vi "Actor Core.vi"(8 "error in":errorcluster, 11 "Root Panel Actor in":refnum<class "Root Panel Actor.lvclass">) -> (0 "error out":errorcluster, 3 "Actor out":refnum<class "Actor.lvclass">)   [LabVIEW 2021, in "Root Panel.lvlib" / "Root Panel Actor.lvclass"]
doc: "The user interface for this panel.\n\n----\nPlease see the following web address for additional documentation and tutorial information:\nhttp://www.mooregoodideas.com/mgi-panel-manager/\n\nAuthor: Derek Trepanier\n\nCopyright (c) 2018, Moore Good Ideas, Inc.\n\nAll rights reserved.\n\nRedistribution and use in source and binary forms, with or without modification, are permitted provided that the following conditions are met:\n\n * Redistributions of source code must retain the above copyright notice, this list of conditions and the following disclaimer.\n * Redistributions in binary form must reproduce the above copyright notice, this list of conditions and the following disclaimer in the documentation and/or other materials provided with the distribution.\n * Neither the name of Moore Good Ideas, Inc. nor the names of its contributors may be used to endorse or promote products derived from this software without specific prior written permission.\n\nTHIS SOFTWARE IS PROVIDED BY THE COPYRIGHT HOLDERS AND CONTRIBUTORS \"AS IS\" AND ANY EXPRESS OR IMPLIED WARRANTIES, INCLUDING, BUT NOT LIMITED TO, THE IMPLIED WARRANTIES OF MERCHANTABILITY AND FITNESS FOR A PARTICULAR PURPOSE ARE DISCLAIMED. IN NO EVENT SHALL THE COPYRIGHT OWNER OR CONTRIBUTORS BE LIABLE FOR ANY DIRECT, INDIRECT, INCIDENTAL, SPECIAL, EXEMPLARY, OR CONSEQUENTIAL DAMAGES (INCLUDING, BUT NOT LIMITED TO, PROCUREMENT OF SUBSTITUTE GOODS OR SERVICES; LOSS OF USE, DATA, OR PROFITS; OR BUSINESS INTERRUPTION) HOWEVER CAUSED AND ON ANY THEORY OF LIABILITY, WHETHER IN CONTRACT, STRICT LIABILITY, OR TORT (INCLUDING NEGLIGENCE OR OTHERWISE) ARISING IN ANY WAY OUT OF THE USE OF THIS SOFTWARE, EVEN IF ADVISED OF THE POSSIBILITY OF SUCH DAMAGE."
uses:
  Root Panel Actor.lvclass
  C:/Program Files (x86)/National Instruments/LabVIEW 2021/vi.lib/MGI/Panel Manager/Panel Actor/Panel Actor/Panel Actor.lvclass
  <vilib>/ActorFramework/Actor/Actor.lvclass
  Root Panel Actor.lvclass/Root Panel Actor.ctl
  <vilib>/ActorFramework/Message Enqueuer/Message Enqueuer.lvclass/Message Enqueuer.ctl
  Appearance Actor/Appearance Actor/Typedefs/User Event-Panel Resize-Data--cluster.ctl
  <vilib>/Utility/miscctls.llb/LVRectTypeDef.ctl
  <vilib>/event_ctls.llb/sizeaction.ctl
  <vilib>/event_ctls.llb/panelstate.ctl
  Appearance Actor/Appearance Actor Messages/User Event-Panel Resize Msg/User Event-Panel Resize Msg.lvclass/User Event-Panel Resize Msg.ctl
  <vilib>/ActorFramework/Message Enqueuer/Enqueue.vi
  <vilib>/ActorFramework/Stop Msg/Stop Msg.lvclass
  C:/Program Files (x86)/National Instruments/LabVIEW 2021/vi.lib/ActorFramework/Message/Message.lvclass
  Appearance Actor/Appearance Actor Messages/User Event-Close-Value Change Msg/User Event-Close-Value Change Msg.lvclass
  Appearance Actor/Appearance Actor Messages/User Event-Maximize-Value Change Msg/User Event-Maximize-Value Change Msg.lvclass
  Appearance Actor/Appearance Actor Messages/User Event-Minimize-Value Change Msg/User Event-Minimize-Value Change Msg.lvclass
  Appearance Actor/Appearance Actor Messages/User Event-Settings-Value Change Msg/User Event-Settings-Value Change Msg.lvclass
  Appearance Actor/Appearance Actor Messages/User Event-Title Bar-Mouse Down Msg/User Event-Title Bar-Mouse Down Msg.lvclass
  Appearance Actor/Appearance Actor Messages/User Event-Panel Resize Msg/User Event-Panel Resize Msg.lvclass
  <vilib>/ActorFramework/Message Priority Queue/Priority Enqueue.vi
  Appearance Actor/Appearance Actor/Appearance Actor.lvclass
  <vilib>/MGI/Panel Manager/Panel Actor/Panel Actor/Panel Actor.lvclass
  <vilib>/MGI/Panel Manager/Panel Actor/Panel Actor Messages/Show Panel Msg/Show Panel Msg.lvclass
  <vilib>/Thomas ALLIBE/Path Utilities/Path Utilities.lvlib
panel:
  in  "Title Bar L":bool
  out "App Icon":picture
  in  "Title Bar M":bool
  out "TB.Title":string
  in  "TB.Dark-Button.Maximize":bool
  in  "TB.Light-Button.Maximize":bool
  in  "TB.Dark-CloseButton":bool
  in  "TB.Light-CloseButton":bool
  in  "TB.Dark-Button.Minimize":bool
  in  "TB.Light-Button.Minimize":bool
  in  "Title Bar R":bool
  in  "SM.Dark-Button.Settings":bool
  in  "SM.Light-Button.Settings":bool
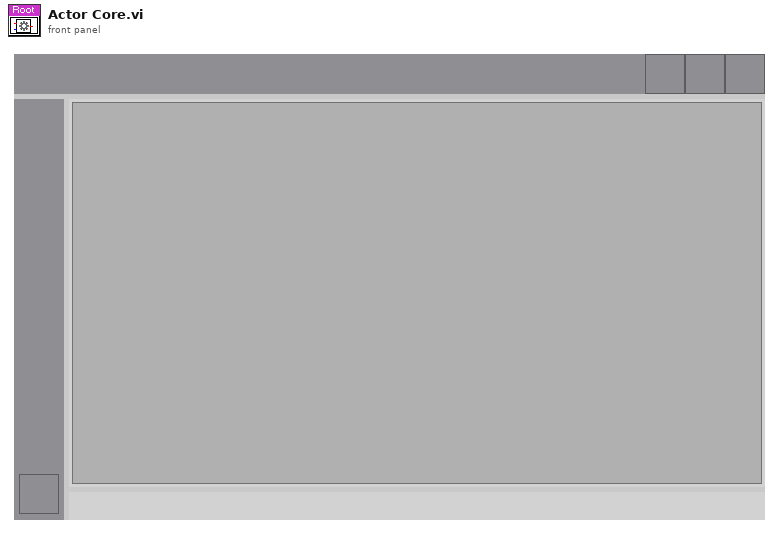
[diagram p1: front panel]
types:
  T1 = cluster{"left":i16, "top":i16, "right":i16, "bottom":i16}
  T2 = typedef "Appearance Actor.lvlib/Appearance Actor.lvclass/User Event-Panel Resize-Data--cluster.ctl" = cluster{"OldBnds":T3, "NewBnds":T3, "Act":T4, "PrevState":T5}
  T3 = typedef "LVRectTypeDef.ctl" = cluster{"Left":i16, "Top":i16, "Right":i16, "Bottom":i16}
  T4 = typedef "sizeaction.ctl" = enum32{"Minimized", "Maximized", "Resized"}
  T5 = typedef "panelstate.ctl" = enum32{"Standard", "Minimized", "Maximized"}
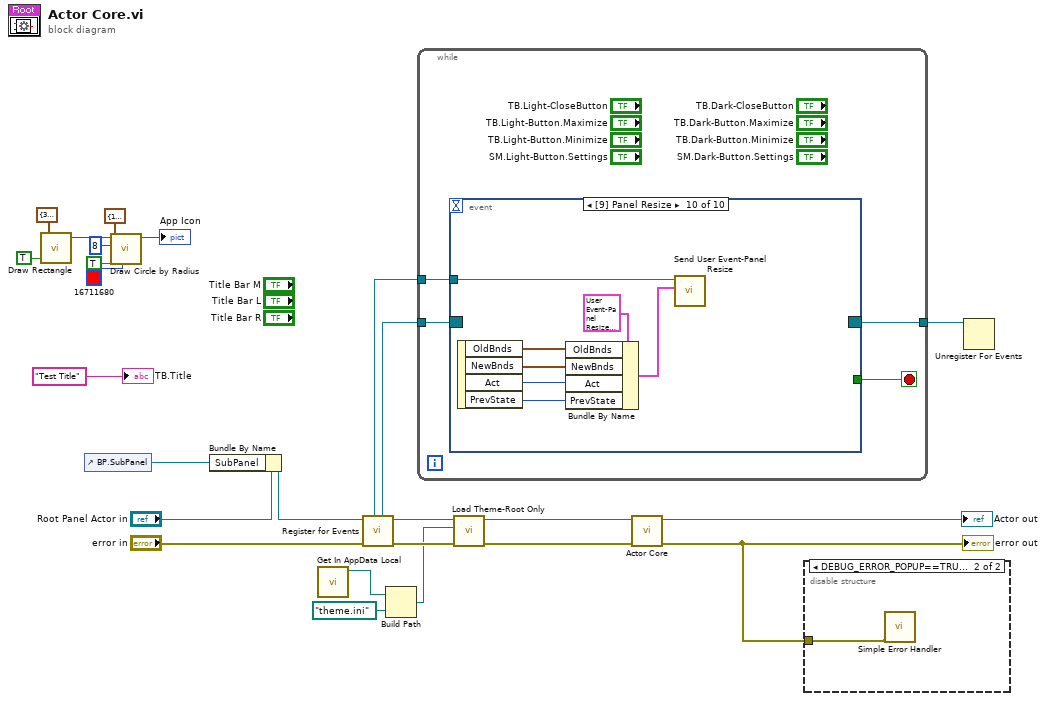
[diagram p0: block diagram]
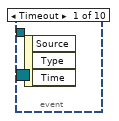
[diagram p3: hidden frame]
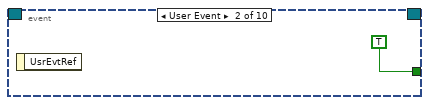
[diagram p4: hidden frame]
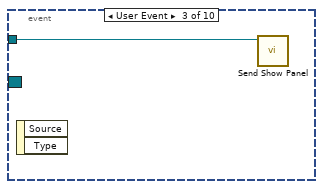
[diagram p5: hidden frame]
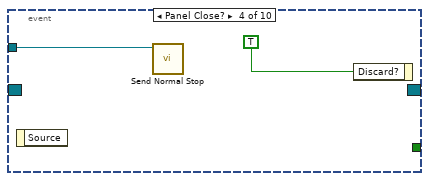
[diagram p6: hidden frame]
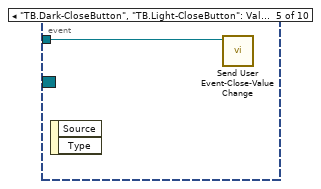
[diagram p7: hidden frame]
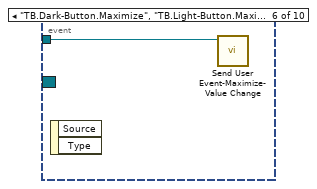
[diagram p8: hidden frame]
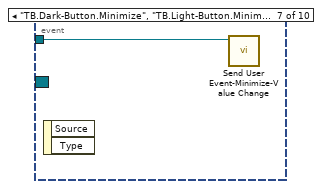
[diagram p9: hidden frame]
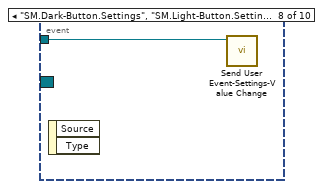
[diagram p10: hidden frame]
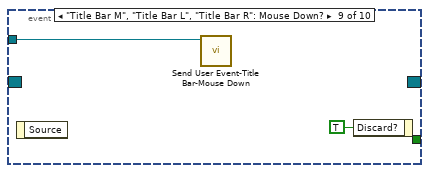
[diagram p11: hidden frame]
diagram:
  n1 = call <vilib>:"Draw Rectangle.vi"("rect"=T1 {"left"=3, "top"=3, "right"=40, "bottom"=30}, "fill?(F)"=TRUE) -> ("new picture"=w19:picture)  [unwired: 7 in]
  n2 = control-ref of="BP.SubPanel"() -> (w2:refnum<vi>)
  n3 = call <vilib>:"Draw Circle by Radius.vi"("color(black)"=u32 16711680, "fill?(F)"=TRUE, "pixel center"=cluster{"horizontal":i16, "vertical":i16} {"horizontal"=15, "vertical"=12}, "radius"=i16 8, "picture"=w19) -> ("new picture"=→"App Icon":picture)  [unwired: 6 in]
  n4 = Bundle By Name(cluster="Root Panel Actor in", "SubPanel"=w2) -> (w4:refnum<class "Root Panel Actor.lvclass">)
  n5 = call <vilib>:"Get In AppData Local.vi"() -> ("Path"=w9:path)  [unwired: 10 in, 1 out]
  n6 = call <vilib>:"Register for Events.vi"("Error In"="error in", "Panel Actor in"=w4) -> ("Error Out"=w11:errorcluster, "Panel Actor out"=w12:refnum<class "Root Panel Actor.lvclass">, "Pnl Actor"=w22:refnum<event-registration>, "Self Enqueuer"=w23:refnum<class "Message Enqueuer.lvclass">)  [unwired: 6 in]
  n7 = Build Path(base path=w9, name or relative path=path "theme.ini") -> (appended path=w7:path)
  n8 = while {
    tunnel: w22 -> [w29]
    tunnel: w23 -> [w28]
    tunnel: [w26] -> w24
    stop <- w27 stop-if-true
    n9 = event shown="[9] Panel Resize" {
      selector: w29 -> [_ _ _ _ _ _ _ _ _ _]
      dyn-events: [_ _ _ _ _ _ _ _ _ _] -> w26
      timeout: _ -> [_ _ _ _ _ _ _ _ _ _]
      tunnel: w28 -> [_ _ w31 w33 w34 w35 w36 w37 w38 w40]
      tunnel: [_ TRUE _ _ _ _ _ _ _ _] -> w27
      event Timeout {
        n10 = event-data() -> ()  [unwired: 1 in, 3 out]
      }
      event User Event {
        n11 = event-data() -> ()  [unwired: 1 in, 1 out]
      }
      event User Event {
        n12 = event-data() -> ()  [unwired: 1 in, 2 out]
        n13 = call <vilib>:"Send Show Panel.vi"("Message Enqueuer in"=w31) -> ()  [unwired: 9 in, 2 out]
      }
      event Panel Close? {
        n14 = event-data() -> ()  [unwired: 1 in, 1 out]
        n15 = call <vilib>:"Send Normal Stop.vi"("Message Enqueuer"=w33) -> ()  [unwired: 10 in, 1 out]
        n16 = event-data("Discard?"=TRUE) -> ()  [unwired: 1 in, 1 out]
      }
      event "TB.Dark-CloseButton", "TB.Light-CloseButton": Value Change {
        n17 = event-data() -> ()  [unwired: 1 in, 2 out]
        n18 = call "Send User Event-Close-Value Change.vi"("Message Enqueuer"=w34) -> ()  [unwired: 9 in, 2 out]
      }
      event "TB.Dark-Button.Maximize", "TB.Light-Button.Maximize": Value Change {
        n19 = event-data() -> ()  [unwired: 1 in, 2 out]
        n20 = call "Send User Event-Maximize-Value Change.vi"("Message Enqueuer"=w35) -> ()  [unwired: 9 in, 2 out]
      }
      event "TB.Dark-Button.Minimize", "TB.Light-Button.Minimize": Value Change {
        n21 = event-data() -> ()  [unwired: 1 in, 2 out]
        n22 = call "Send User Event-Minimize-Value Change.vi"("Message Enqueuer"=w36) -> ()  [unwired: 9 in, 2 out]
      }
      event "SM.Dark-Button.Settings", "SM.Light-Button.Settings": Value Change {
        n23 = event-data() -> ()  [unwired: 1 in, 2 out]
        n24 = call "Send User Event-Settings-Value Change.vi"("Message Enqueuer"=w37) -> ()  [unwired: 9 in, 2 out]
      }
      event "Title Bar M", "Title Bar L", "Title Bar R": Mouse Down? {
        n25 = event-data() -> ()  [unwired: 1 in, 1 out]
        n26 = call "Send User Event-Title Bar-Mouse Down.vi"("Message Enqueuer"=w38) -> ()  [unwired: 9 in, 2 out]
        n27 = event-data("Discard?"=TRUE) -> ()  [unwired: 1 in, 1 out]
      }
      event Panel Resize {
        n28 = event-data() -> ("OldBnds"=w44:T3, "NewBnds"=w43:T3, "Act"=w42:T4, "PrevState"=w41:T5)  [unwired: 1 in]
        n29 = Bundle By Name(cluster=T2 {"OldBnds"={"Left"=0, "Top"=0, "Right"=0, "Bottom"=0}, "NewBnds"={"Left"=0, "Top"=0, "Right"=0, "Bottom"=0}, "Act"=enum."Resized", "PrevState"=enum."Standard"} ("Panel Resize Data"), "OldBnds"=w44, "NewBnds"=w43, "Act"=w42, "PrevState"=w41) -> (w46:T2)
        n30 = call "Send User Event-Panel Resize.vi"("Panel Resize Data"=w46, "Message Enqueuer"=w40) -> ()  [unwired: 8 in, 2 out]
      }
    }
  }
  n31 = call-dynamic "Load Theme-Root Only.vi"("Error In"=w11, "Theme File Path"=w7, "Appearance Actor in"=w12) -> ("Error Out"=w6:errorcluster, "Appearance Actor out"=w10:refnum<class "Root Panel Actor.lvclass">)  [unwired: 7 in]
  n32 = call-parent "Actor Core.vi"("error in"=w6, "Appearance Actor in"=w10) -> ("error out"=w1:errorcluster, "Actor out"=→"Actor out":refnum<class "Actor.lvclass">)  [unwired: 8 in]
  "error out" <- w1
  n33 = disable-structure shown="DEBUG_ERROR_POPUP==TRUE" {
    disable-tunnel: w1 -> [_ w47]
    frame condition #0 {
    }
    frame condition #1 (active) {
      n34 = call <vilib>:"Simple Error Handler.vi"("error in (no error)"=w47) -> ()  [unwired: 4 in, 5 out]
    }
  }
  n35 = Unregister For Events(event registration refnum=w24) -> ()  [unwired: 1 in, 1 out]
  "TB.Title" <- "Test Title" ("Title")
